vi "Read LabVIEW Info.vi"() -> (0 "error out":errorcluster, 2 "LabVIEW Path":path, 3 "VI Server Port":u16)   [LabVIEW 2024, in "Wordle Scorer.lvlib"]
uses:
  Wordle Scorer.lvlib
  <vilib>/Utility/config.llb/Read Key (U32).vi
  <vilib>/Utility/config.llb/Read Key (Path).vi
  <vilib>/Utility/config.llb/NI_LVConfig.lvlib
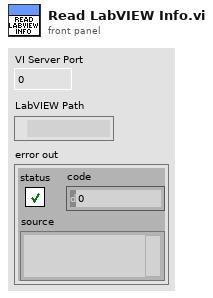
[diagram p1: front panel]
types:
  T1 = typedef "NI_LVConfig.lvlib/Config Data RefNum.ctl" = refnum<k1>
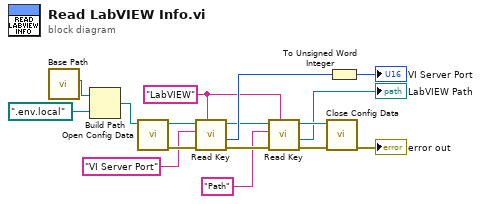
[diagram p0: block diagram]
diagram:
  w3 = "LabVIEW" ("section")
  n1 = call "Base Path.vi"() -> ("Base Path"=w16:path)  [unwired: 11 in]
  n2 = Build Path(base path=w16, name or relative path=path ".env.local") -> (appended path=w14:path)
  n3 = call <vilib>:"Open Config Data.vi"("configuration file path"=w14) -> ("error out"=w13:errorcluster, "refnum"=w12:T1)  [unwired: 8 in, 1 out]
  n4 = call-poly <vilib>:"Read Key.vi"("section"=w3, "error in (no error)"=w13, "key"="VI Server Port", "refnum"=w12) -> ("error out"=w6:errorcluster, "value"=w9:u32, "refnum out"=w7:T1)  [unwired: 4 in, 1 out]
  n5 = call-poly <vilib>:"Read Key.vi"("section"=w3, "error in (no error)"=w6, "key"="Path", "refnum"=w7) -> ("error out"=w4:errorcluster, "value"=→"LabVIEW Path":path, "refnum out"=w5:T1)  [unwired: 4 in, 1 out]
  n6 = call <vilib>:"Close Config Data.vi"("error in (no error)"=w4, "refnum"=w5) -> ("error out"=→"error out":errorcluster)  [unwired: 8 in, 1 out]
  n7 = To Unsigned Word Integer(number=w9) -> (unsigned 16bit integer=→"VI Server Port":u16)
